vi "DAQmx Timing (Pipelined Sample Clock).vi"(0 "task/channels in":refnum<k21>, 1 "sample mode":i32(ring)=10178 items=["Finite Samples"=10178, "Continuous Samples"=10123, "Hardware Timed Single Point"=12522], 2 "samples per channel":i32=1000, 5 "rate":dbl=1000.0 format="%0.2f", 7 "source":tag, 9 "active edge":i32(ring)=10280 items=["Rising"=10280, "Falling"=10171], 11 "error in":errorcluster) -> (4 "task out":refnum<k21>, 15 "error out":errorcluster)   [LabVIEW 2020]
doc: "Sets the source of the Sample Clock, the rate of the Sample Clock, and the number of samples to acquire or generate. The device acquires or generates samples on each Sample Clock edge, but it does not respond to certain triggers until a few Sample Clock edges later. Pipelining allows higher data transfer rates at the cost of increased trigger response latency. Refer to the device documentation for information about which triggers pipelining affects.\n\nThis timing type allows handshaking using the Pause trigger and either the Ready for Transfer event or the Data Active event. Refer to the device documentation for more information.\n\nThis timing type is supported only by the NI 6536 and NI 6537."
uses:
  nilvaiu.dll
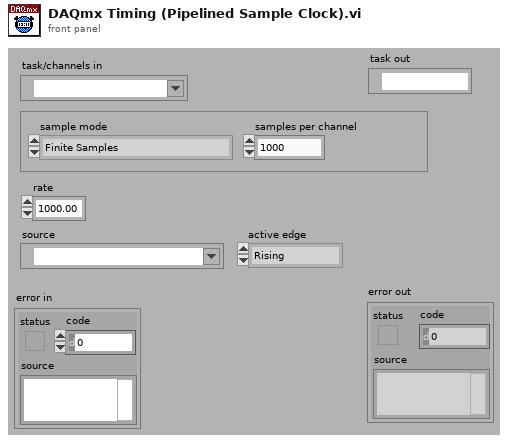
[diagram p1: front panel]
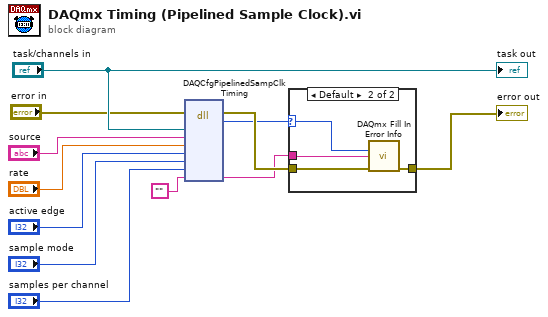
[diagram p0: block diagram]
diagram:
  n1 = dll-call lib="nilvaiu.*" fn="DAQCfgPipelinedSampClkTiming"(error in="error in", "taskID"="task/channels in", "source"="source", "rate"="rate", "activeEdge"="active edge", "sampleMode"="sample mode", "samplesPerChannel"="samples per channel", "extendedErrorInfo"="") -> (error out=w10:errorcluster, "return type"=w8:i32, "extendedErrorInfo"=w9:string)  [unwired: 4 in, 5 out]
  n2 = case shown="Default" w8 {
    selector: w8 -> [_ w15]
    tunnel: w10 -> [w13 w17]
    tunnel: [w13 w16] -> w12
    tunnel: w9 -> [_ w14]
    frame 0 {
    }
    frame Default {
      n3 = call "DAQmx Fill In Error Info.vi"("status code"=w15, "extended error info"=w14, "error in"=w17) -> ("error out"=w16:errorcluster)  [unwired: 1 in, 11 out]
    }
  }
  "error out" <- w12
  "task out" <- "task/channels in"
